vi "CRYFlatten Graph Property.vi"(10 "Cluster Name":string, 11 "GraphProperty":string) -> (3 "GraphProperty Flattened":string)   [LabVIEW 2013]
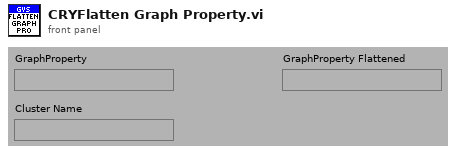
[diagram p1: front panel]
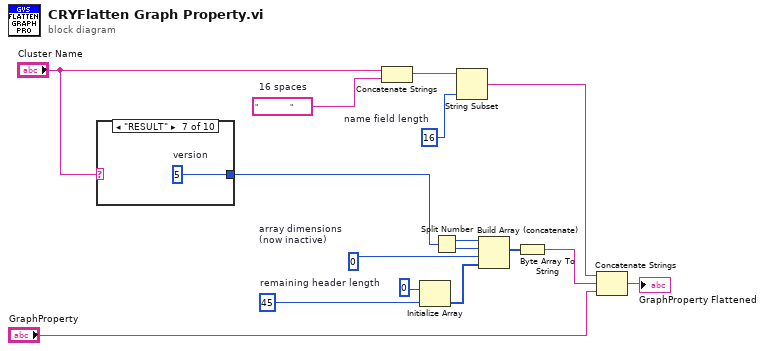
[diagram p0: block diagram]
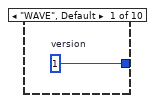
[diagram p2: hidden frame]
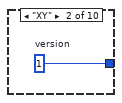
[diagram p3: hidden frame]
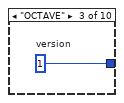
[diagram p4: hidden frame]
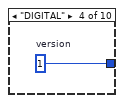
[diagram p5: hidden frame]
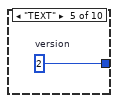
[diagram p6: hidden frame]
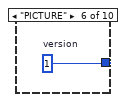
[diagram p7: hidden frame]
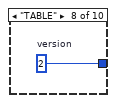
[diagram p8: hidden frame]
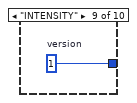
[diagram p9: hidden frame]
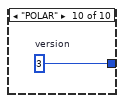
[diagram p10: hidden frame]
diagram:
  w4 = u8 0  # array dimensions (now inactive)
  w7 = 16  # name field length
  w8 = "                "  # 16 spaces
  w13 = 45  # remaining header length
  n1 = case shown="\"RESULT\"" "Cluster Name" {
    tunnel: [w17 w18 w19 w20 w21 w22 w23 w24 w25 w26] -> w1
    frame "WAVE", Default {
      w17 = u16 1  # version
    }
    frame "XY" {
      w18 = u16 1  # version
    }
    frame "OCTAVE" {
      w19 = u16 1  # version
    }
    frame "DIGITAL" {
      w20 = u16 1  # version
    }
    frame "TEXT" {
      w21 = u16 2  # version
    }
    frame "PICTURE" {
      w22 = u16 1  # version
    }
    frame "RESULT" {
      w23 = u16 5  # version
    }
    frame "TABLE" {
      w24 = u16 2  # version
    }
    frame "INTENSITY" {
      w25 = u16 1  # version
    }
    frame "POLAR" {
      w26 = u16 3  # version
    }
  }
  n2 = Concatenate Strings("Cluster Name", w8) -> (w6:string)
  n3 = Initialize Array(u8 0, w13) -> (w9:u8[])
  n4 = Split Number(x=w1) -> (hi(x)=w16:u8, lo(x)=w15:u8)
  n5 = String Subset(string=w6, length (rest)=w7) -> (substring=w5:string)  [unwired: 1 out]
  n6 = Build Array (concatenate)(w16, w15, w4, w9) -> (w12:u8[])
  n7 = Byte Array To String(unsigned byte array=w12) -> (string=w10:string)
  n8 = Concatenate Strings(w5, w10, "GraphProperty") -> (→"GraphProperty Flattened":string)
